vi "FPGA.vi"() -> ()   [LabVIEW 2017]
uses:
  <vilib>/Platform/TimedLoop/XDataNode/timing_clust.ctl
  <vilib>/Platform/TimedLoop/XDataNode/nitl_modes.ctl
  <vilib>/Platform/TimedLoop/XDataNode/wakeup.ctl
  <vilib>/rvi/FXPMathLib/basic elements/FxpIntAccumulator/subVIs/nifxpmath_IntAccumulator_SimConfig.ctl
  <vilib>/rvi/Emulation/niFpgaGetClockAttributes.vi
  <vilib>/rvi/Emulation/niFpgaSctlEmulationGetInTimedLoop.vi
  <vilib>/rvi/Emulation/niFpgaEmulationReportErrorSimple.vi
  <vilib>/rvi/Emulation/niFpgaEmulationIsFPGAContextNoSignature.vi
  <vilib>/rvi/DataTransferAndStorage/Container/Common/niFpgaContainerGetUniqueNameForEmu.vi
  <vilib>/rvi/Memory/Memory_Emulation/niFpgaMemoryEmulationCacheClearOnFirstRun.vi
  <vilib>/rvi/Memory/Memory_Emulation/nirvimemoryEmulationManagerCache_MakeExclusive.vi
  <vilib>/rvi/Memory/Memory_Emulation/niFpgaMemoryEmulationValidateCache.vi
  <vilib>/rvi/Memory/Memory_Emulation/nirvimemoryEmulationManagerCache_InsertValue.vi
  <vilib>/Utility/error.llb/Clear Errors.vi
  <vilib>/rvi/Memory/Memory_Emulation/nirvimemoryEmulationManagerCache_ReleaseExclusive.vi
  <vilib>/rvi/Memory/Memory_Emulation/nirvimemoryEmulationManagerCache_GetValue.vi
  <vilib>/rvi/Memory/Memory_Emulation/nirvimemoryEmulationManagerCache_SetValue.vi
  <vilib>/rvi/Emulation/niFpgaProcessEmulError.vi
  <vilib>/rvi/Emulation/niFpgaCriticalErrorInLSC.vi
  <vilib>/rvi/interface/RandomDataEmulation/niFpgaRandomDataHandleErrors.vi
  <vilib>/rvi/Analysis/common/codeGenErrors/XNode/niFpgaXNodeCodeGenErrorHandle.vi
  <vilib>/rvi/FXPMathLib/basic elements/FxpIntAccumulator/simVIs/DllFxpIntAccumulator_sub.vi
  <vilib>/rvi/eio/common/nirviEmuTemplateMethod_errors.vi
  <vilib>/Platform/TimedLoop/XDataNode/XDataNode.xnode
  <vilib>/rvi/DataTransferAndStorage/Container/XNode/niFpgaContainer.xnode
  <vilib>/rvi/DataTransferAndStorage/Register/Emulation/niFpgaRegisterEmulation.vi
  <vilib>/rvi/interface/RandomDataEmulation/nirviRandomDataFpgaReadWriteTemplate.vi
  <vilib>/rvi/Analysis/measure/mean-var-std/XNode/niFpgaMean-Var-Std.xnode
  <vilib>/rvi/FXPMathLib/basic elements/FxpIntAccumulator/XNode/nifxpmath_IntAccumulator.xnode
  <vilib>/eio/EIONode/EIONode.xnode
  <vilib>/Platform/TimedLoop/XDataNode/XDNodeRunTimeDep.lvlib
panel:
  in  "White Noise Data Length":u32
  out "Chassis Temperature":i16
  out "4-Element Average":i32
  in  "User Fpga Led":u8
  out "White Noise Data Timeout?":bool
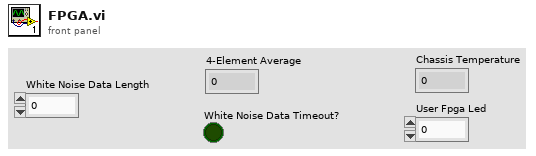
[diagram p1: front panel]
types:
  T1 = typedef "XDNodeRunTimeDep.lvlib/timing_clust.ctl" = cluster{"Expected End [f-1]":u64, "Actual End [f-1]":u64, "Finished Late? [f-1]":bool, "Expected End [i-1]":u64, "Actual End [i-1]":u64, "Finished Late? [i-1]":bool, "Expected Start [i]":u64, "Actual Start [i]":u64, "Expected Start [f]":u64, "Actual Start [f]":u64, "Source Name":string, "Structure Name":string, "Period":i64, "Deadline":i64, "Offset":i64, "Start":i64, "Priority":i32, "Timeout":i32, "Mode":T2, "Wakeup Reason":T3, "Error":errorcluster, "Source Type":string, "Secondary Source Type":string, "Global End Time":u64, "Global Start Time":u64, "Frame Duration":u64, "Iteration Duration":u64, "Assigned CPU":i32, "I/O Scan Engine Mode":u32}
  T2 = typedef "XDNodeRunTimeDep.lvlib/nitl_modes.ctl" = enum32{"No Change", "Process missed periods, maintain original phase", "Discard missed periods, maintain original phase", "Process missed periods, ignore original phase", "Discard missed periods, ignore original phase"}
  T3 = typedef "XDNodeRunTimeDep.lvlib/wakeup.ctl" = enum32{"Normal", "Aborted", "Asynchronous wakeup", "Timing source error", "Timed loop error", "Timeout"}
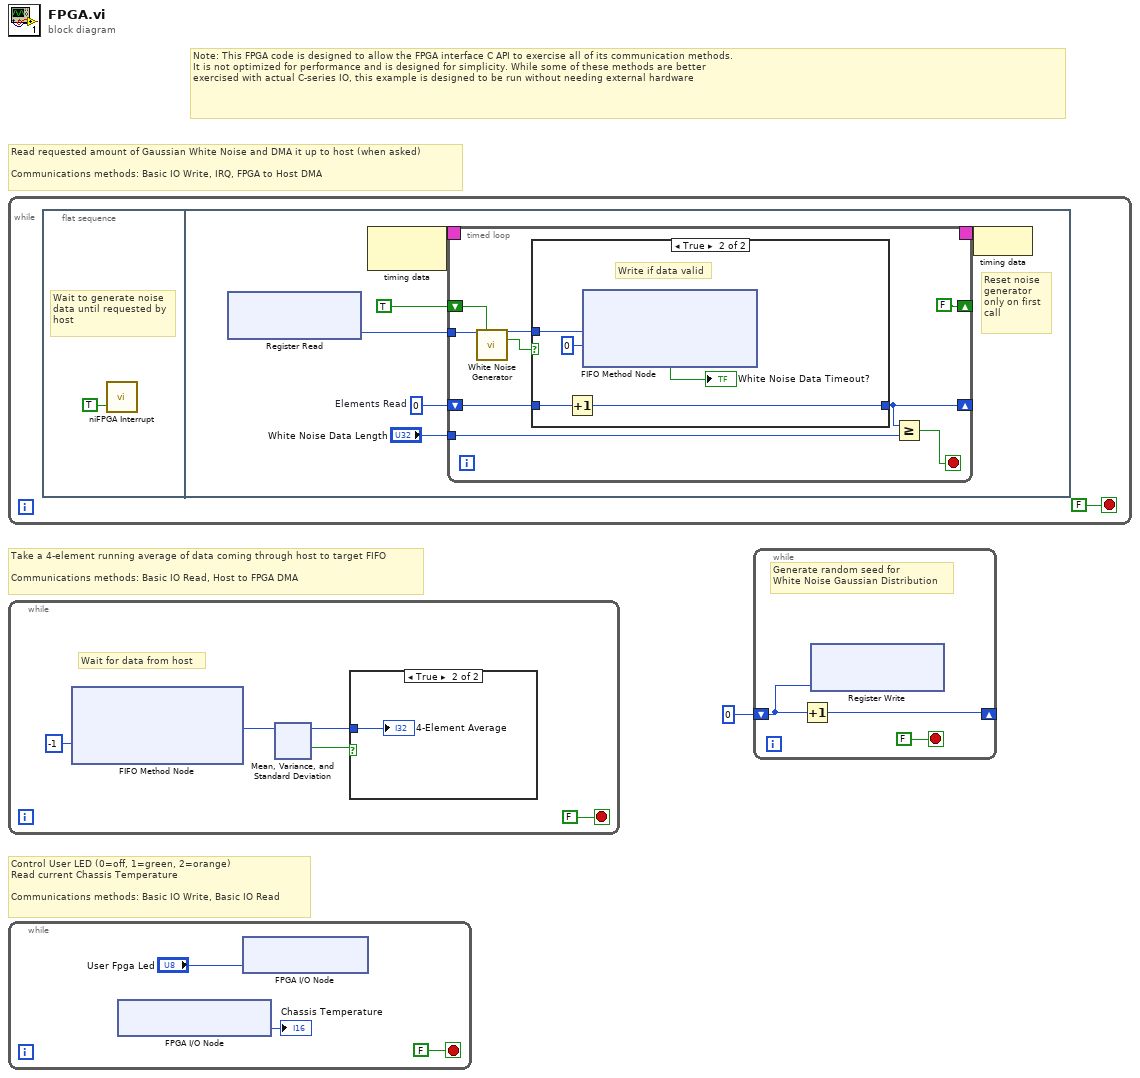
[diagram p0: block diagram]
diagram:
  # "Note: This FPGA code is designed to allow the FPGA interface C API to exercise all of its communication methods. \nIt is not optimized for performance and is designed for simplicity. While some of these methods are better\nexercised with actual C-series IO, this example is designed to be run without needing external hardware"
  # "Control User LED (0=off, 1=green, 2=orange)\nRead current Chassis Temperature\n\nCommunications methods: Basic IO Write, Basic IO Read"
  # "Take a 4-element running average of data coming through host to target FIFO\n\nCommunications methods: Basic IO Read, Host to FPGA DMA"
  # "Read requested amount of Gaussian White Noise and DMA it up to host (when asked)\n\nCommunications methods: Basic IO Write, IRQ, FPGA to Host DMA"
  n1 = while {
    stop <- FALSE stop-if-true
    n2 = flat-sequence {
      frame #0 {
        # "Wait to generate noise\ndata until requested by\nhost"
        n3 = call <vilib>:"niFPGA Interrupt.vi"("Wait Until Cleared (F)"=TRUE) -> ()  [unwired: 2 in]
      }
      frame #1 {
        w4 = u32 0  # Elements Read
        # "Reset noise \ngenerator\nonly on first \ncall"
        n4 = xnode "Register Read"() -> ("Data"=w7:u32)  [unwired: 1 in, 1 out]
        n5 = node-c288() -> (w9:T1)  [unwired: 1 in]
        n6 = timed-loop {
          timing: w9 -> [_]
          timing-out: [_] -> w8
          tunnel: w7 -> [w16]
          shift-right: [FALSE ("reset")] -> _
          shift-left: TRUE ("reset") -> [w15]
          tunnel: "White Noise Data Length" -> [w11]
          shift-right: [w12] -> _
          shift-left: w4 -> [w13]
          stop <- w10 stop-if-true
          n7 = call "White Noise Generator"("seed"=w16, "reset"=w15) -> ("white noise out"=w18:i16, "data valid?"=w17:bool)  [unwired: 12 in]
          n8 = case shown="True" w17 {
            tunnel: w18 -> [_ w22]
            tunnel: w13 -> [w19 w21]
            tunnel: [w19 w20] -> w12
            frame False {
              # "Don't write if data invalid"
            }
            frame True {
              # "Write if data valid"
              n9 = Increment(x=w21) -> (x+1=w20:u32)
              n10 = xnode ("FIFO Method Node")("Element"=w22, "Timeout"=0) -> ("Timed Out?"=→"White Noise Data Timeout?":bool)  [unwired: 1 in, 1 out]
            }
          }
          n11 = Greater Or Equal?(x=w12, y=w11) -> (x >= y?=w10:bool)
        }
        n12 = node-c288(w8) -> ()
      }
    }
  }
  n13 = while {
    stop <- FALSE stop-if-true
    # "Wait for data from host"
    n14 = xnode ("FIFO Method Node")("Timeout"=-1) -> ("Element"=w31:i32)  [unwired: 1 in, 2 out]
    n15 = xnode "Mean, Variance, and Standard Deviation"("input data"=w31) -> ("mean"=w30:i32, "output valid"=w29:bool)  [unwired: 1 in]
    n16 = case shown="True" w29 {
      tunnel: w30 -> [_ w115]
      frame False {
        # "Not enough samples"
      }
      frame True {
        "4-Element Average" <- w115
      }
    }
  }
  n17 = while {
    stop <- FALSE stop-if-true
    n18 = xnode "FPGA I/O Node"() -> ("Chassis Temperature"=→"Chassis Temperature":i16)  [unwired: 1 in, 1 out]
    n19 = xnode "FPGA I/O Node"("USER FPGA LED"="User Fpga Led") -> ()  [unwired: 1 in, 1 out]
  }
  n20 = while {
    shift-right: [w119] -> _
    shift-left: u32 0 ("Sinewave Frequency") -> [w120]
    stop <- FALSE stop-if-true
    # "Generate random seed for\nWhite Noise Gaussian Distribution"
    n21 = Increment(x=w120) -> (x+1=w119:u32)
    n22 = xnode "Register Write"("Data"=w120) -> ()  [unwired: 1 in, 1 out]
  }
